vi "ReadFuzzyMap.vi"(7 "error in (no error)":errorcluster, 10 "VISA in":refnum<visa-resource-name>) -> (0 "error out":errorcluster, 2 "Table Control":string[][](table), 3 "VISA out":refnum<visa-resource-name>)   [LabVIEW 2016]
uses:
  <vilib>/NI Modbus.llb/MB Serial Master Query Read Holding Registers (poly).vi
panel:
  out "Exception Code":u8 format="%.0x"
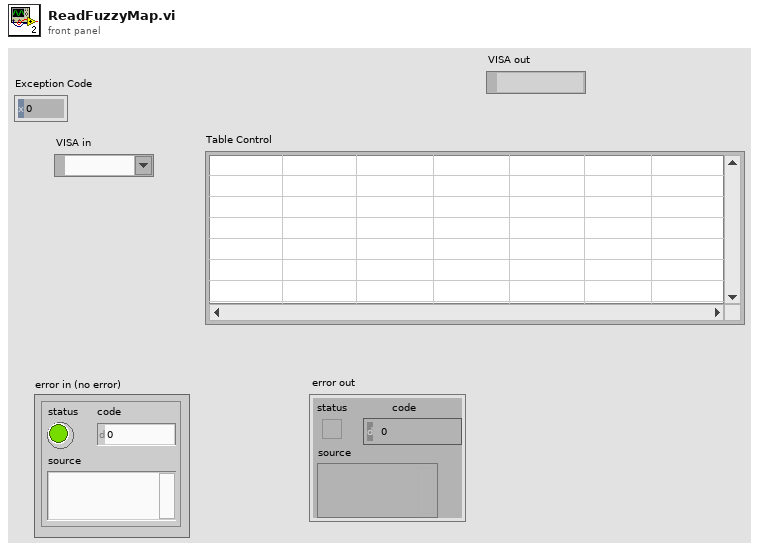
[diagram p1: front panel]
types:
  T1 = cluster{"Mode":enum16{"RTU", "ASCII"}, "Slave Address":u8}
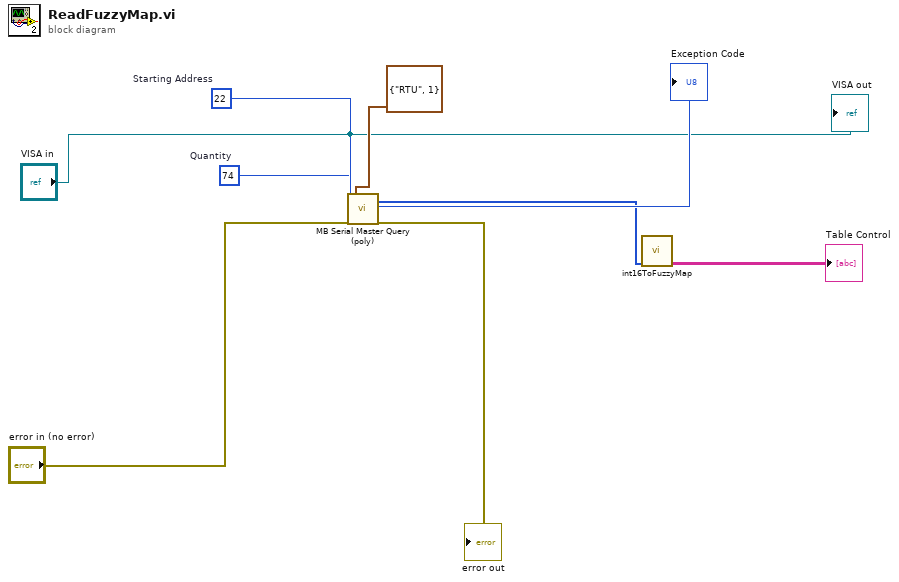
[diagram p0: block diagram]
diagram:
  w8 = u16 74  # Quantity
  w9 = u16 22  # Starting Address
  n1 = call-poly <vilib>:"MB Serial Master Query (poly).vi"("VISA resource name"="VISA in", "Starting Address"=w9, "Quantity"=w8, "error in"="error in (no error)", "Serial Parameters"=T1 {"Mode"=enum."RTU", "Slave Address"=1}) -> ("Holding Registers"=w3:u16[], "Exception Code"=→"Exception Code":u8, "error out"=→"error out":errorcluster)  [unwired: 11 in, 1 out]
  n2 = call "int16ToFuzzyMap.vi"("Input Registers"=w3) -> ("Table Control"=→"Table Control":string[][])  [unwired: 10 in]
  "VISA out" <- "VISA in"
